vi "Test Full API Test Coverage.vi"(8 "error in (no error)":errorcluster) -> (0 "error out":errorcluster)   [LabVIEW 2013, in "TEST JKI State Machine API.lvlib"]
uses:
  TEST JKI State Machine API.lvlib
  <vilib>/addons/_JKI Toolkits/Caraya/classes/Test/Test.lvclass
  <vilib>/addons/_JKI Toolkits/Caraya/classes/Assert/Assert.lvclass
panel:
  out "Untested VIs":string[](array[string])
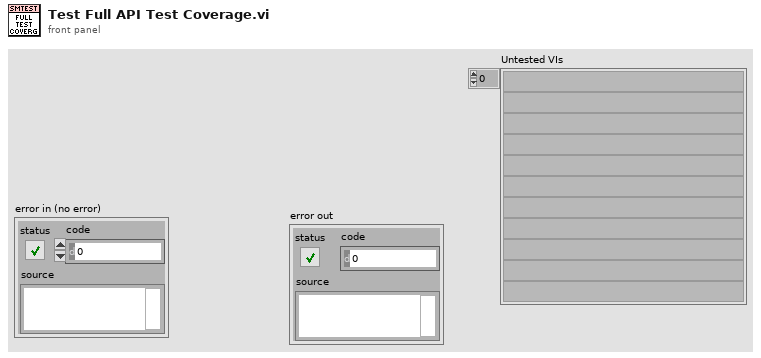
[diagram p1: front panel]
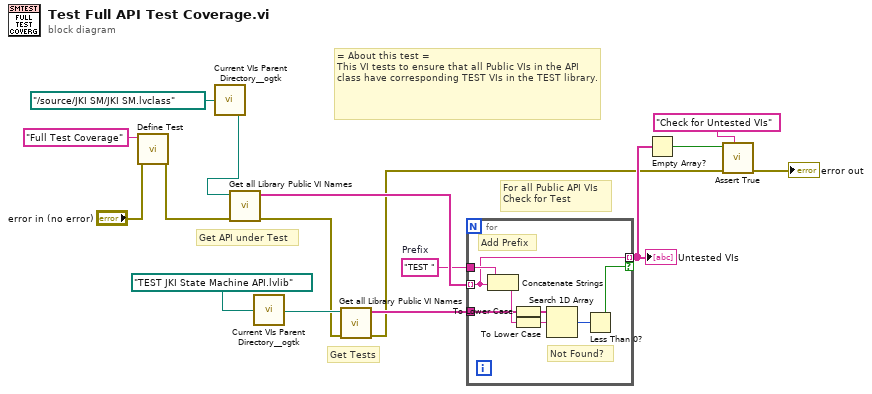
[diagram p0: block diagram]
diagram:
  w15 = "TEST "  # Prefix
  # "= About this test =\nThis VI tests to ensure that all Public VIs in the API class have corresponding TEST VIs in the TEST library."
  # "For all Public API VIs\nCheck for Test"
  # "Get Tests"
  # "Get API under Test"
  n1 = call <vilib>:"Define Test.vi"("error in (no error)"="error in (no error)", "Label (VI Title)"="Full Test Coverage") -> ("error out"=w6:errorcluster)  [unwired: 9 in]
  n2 = call <userlib>:"Current VIs Parent Directory__ogtk.vi"("Relative path (.)"=path "../source/JKI SM/JKI SM.lvclass") -> ("Parent Directory (+ Relative)"=w12:path)  [unwired: 4 in]
  n3 = call "Get all Library Public VI Names.vi"("error in (no error)"=w6, "Library or Class Path"=w12) -> ("error out"=w9:errorcluster, "Public VI Names"=w16:string[])  [unwired: 8 in]
  n4 = call <userlib>:"Current VIs Parent Directory__ogtk.vi"("Relative path (.)"=path "TEST JKI State Machine API.lvlib" ("Path")) -> ("Parent Directory (+ Relative)"=w10:path)  [unwired: 4 in]
  n5 = call "Get all Library Public VI Names.vi"("error in (no error)"=w9, "Library or Class Path"=w10) -> ("error out"=w3:errorcluster, "Public VI Names"=w14:string[])  [unwired: 8 in]
  n6 = for {
    tunnel: w16 -> [w20] mode=indexing
    tunnel: w15 -> [w24]
    tunnel: w14 -> [w22]
    tunnel: [w20] -> w5 mode=indexing if=w19
    # "Add Prefix"
    # "Not Found?"
    n7 = Concatenate Strings(w24, w20) -> (w23:string)
    n8 = To Lower Case(string=w22) -> (all lower case string=w18:string[])
    n9 = To Lower Case(string=w23) -> (all lower case string=w17:string)
    n10 = Search 1D Array(1D array=w18, element=w17) -> (index of element=w21:i32)  [unwired: 1 in]
    n11 = Less Than 0?(x=w21) -> (x < 0?=w19:bool)
  }
  "Untested VIs" <- w5
  n12 = Empty Array?(array=w5) -> (empty?=w4:bool)
  n13 = call <vilib>:"Assert True.vi"("Label"="Check for Untested VIs", "error in (no error)"=w3, "True?"=w4) -> ("error out"=→"error out":errorcluster)  [unwired: 8 in]
